vi "ImageReBlock_32to64 (子VI).vi"(1 "BlockImg":dbl[][][](array[numeric])) -> (0 "ReBlockImg":dbl[][](array[numeric]))   [LabVIEW 2018]
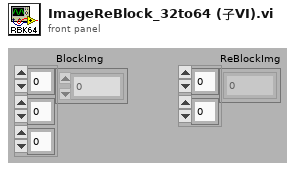
[diagram p1: front panel]
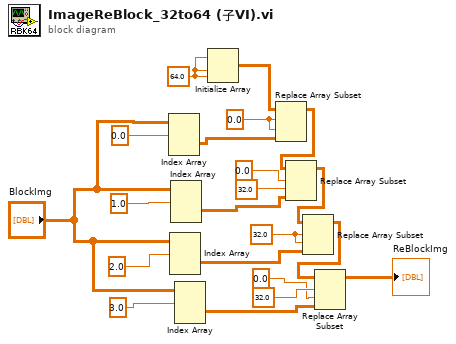
[diagram p0: block diagram]
diagram:
  w2 = 32.0 ("size (default 128)")
  w16 = 0.0
  w18 = 64.0 ("size (default 128)")
  n1 = Index Array(array="BlockImg", index (dim 0)=0.0) -> (element=w14:dbl[][])  [unwired: 2 in]
  n2 = Index Array(array="BlockImg", index (dim 0)=2.0) -> (element=w7:dbl[][])  [unwired: 2 in]
  n3 = Index Array(array="BlockImg", index (dim 0)=1.0) -> (element=w8:dbl[][])  [unwired: 2 in]
  n4 = Index Array(array="BlockImg", index (dim 0)=3.0) -> (element=w6:dbl[][])  [unwired: 2 in]
  n5 = Initialize Array(w18, w18, w18) -> (w17:dbl[][])
  n6 = Replace Array Subset(array=w17, new element=w14, index (row)=w16, index (col)=w16) -> (w10:dbl[][])
  n7 = Replace Array Subset(array=w10, new element=w8, index (row)=0.0, index (col)=32.0 ("size (default 128)")) -> (w5:dbl[][])
  n8 = Replace Array Subset(array=w5, new element=w7, index (row)=w2, index (col)=w2) -> (w20:dbl[][])
  n9 = Replace Array Subset(array=w20, new element=w6, index (row)=32.0 ("size (default 128)"), index (col)=0.0) -> (→"ReBlockImg":dbl[][])
